vi "BoxI32.vi"(10 "Numeric":i32) -> (2 "I32 out":refnum<class "I32.lvclass">)   [LabVIEW 2013, in "LapDog.Collections.v1.Common.lvlib" / "I32.lvclass"]
uses:
  I32.lvclass
  I32.lvclass/I32.ctl
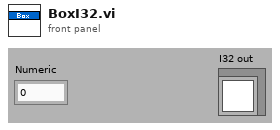
[diagram p1: front panel]
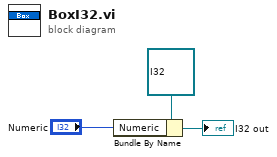
[diagram p0: block diagram]
diagram:
  n1 = Bundle By Name(cluster=refnum<class "I32.lvclass"> refnum ("LapDog.Collections.v0.Lists.Interfaces.lvlib:String.lvclass"), "Numeric"="Numeric") -> (→"I32 out":refnum<class "I32.lvclass">)
